vi "MeasureSTARTTime.vi"(8 "error in":errorcluster, 10 "Timeout / ms":u32=1000, 11 "VISA resource name":refnum<visa-resource-name>) -> (0 "error out":errorcluster, 1 "Local time":timestamp, 2 "System time / us":u32=437417, 3 "VISA resource name out":refnum<visa-resource-name>)   [LabVIEW 2017, in "GP22_TDC_Arduinoed.lvlib"]
doc: "Measure the time of arrival of the next pulse at the START input, in milliseconds since the unit was last reset. The counter rolls over every 24 hours."
uses:
  GP22_TDC_Arduinoed.lvlib
  <vilib>/ErrorRing/Error Ring.xnode
  <vilib>/Utility/error.llb/Error Cluster From Error Code.vi
  <vilib>/regexp/Match Regular Expression.xnode
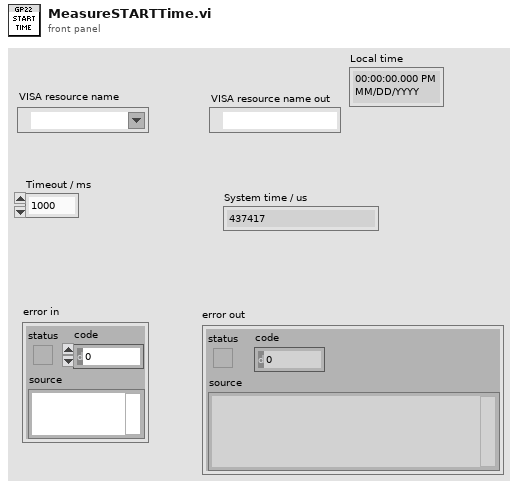
[diagram p1: front panel]
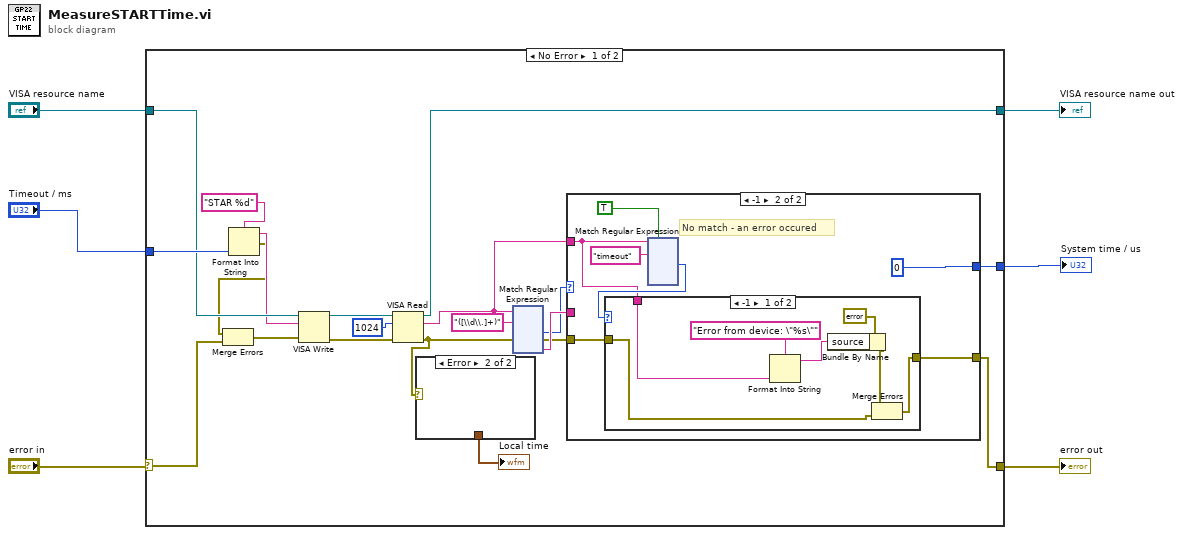
[diagram p0: block diagram]
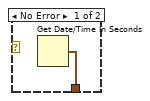
[diagram p2: hidden frame]
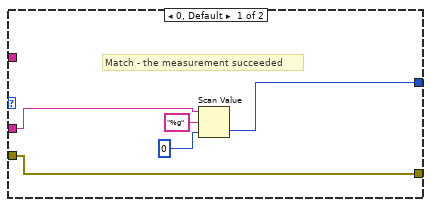
[diagram p3: hidden frame]
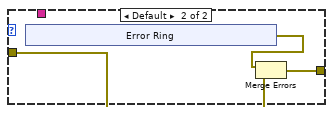
[diagram p4: hidden frame]
diagram:
  n1 = case shown="No Error" "error in" {
    selector: "error in" -> [w20 w288]
    tunnel: "VISA resource name" -> [w24 w287]
    tunnel: [w16 w287] -> w5
    tunnel: [w15 w288] -> w4
    tunnel: "Timeout / ms" -> [w25 _]
    tunnel: [w14 _] -> w1
    frame No Error {
      n2 = Format Into String(format string="STAR %d", w25) -> (resulting string=w23:string, error out=w21:errorcluster)  [unwired: 2 in]
      n3 = Merge Errors(w21, w20) -> (w22:errorcluster)
      n4 = VISA Write(VISA resource name=w24, write buffer=w23, error in (no error)=w22) -> (VISA resource name out=w18:refnum<visa-resource-name>, error out=w19:errorcluster)  [unwired: 1 out]
      n5 = VISA Read(VISA resource name=w18, byte count=u32 1024, error in (no error)=w19) -> (VISA resource name out=w16:refnum<visa-resource-name>, read buffer=w9:string, error out=w8:errorcluster)  [unwired: 1 out]
      n6 = case shown="Error" w8 {
        tunnel: [w27 _] -> w7
        frame No Error {
          n7 = Get Date/Time In Seconds() -> (seconds since 1Jan1904=w27:timestamp)
        }
        frame Error {
        }
      }
      "Local time" <- w7
      n8 = xnode "Match Regular Expression"("input string"=w9, "regular expression"="([\\d\\.]+)", "error in"=w8) -> ("offset past match"=w11:i32, "error out"=w10:errorcluster, "submatch 1"=w12:string)  [unwired: 3 in, 3 out]
      n9 = case shown="-1" w11 {
        tunnel: w10 -> [w145 w154]
        tunnel: [w145 w155] -> w15
        tunnel: w12 -> [w147 _]
        tunnel: [w146 u32 0] -> w14
        tunnel: w9 -> [_ w149]
        frame 0, Default {
          # "Match - the measurement succeeded"
          n10 = Scan Value(string=w147, format string="%g", default (0 dbl)=u32 0) -> (value=w146:u32)  [unwired: 1 out]
        }
        frame -1 {
          # "No match - an error occured"
          n11 = xnode "Match Regular Expression"("input string"=w149, "regular expression"="timeout", "ignore case? (F)"=TRUE) -> ("offset past match"=w150:i32)  [unwired: 3 in, 5 out]
          n12 = case shown="-1" w150 {
            tunnel: [w159 w165] -> w155
            tunnel: w154 -> [w158 w163]
            tunnel: w149 -> [w156 _]
            frame -1 {
              n13 = Format Into String(format string="Error from device: \"%s\"", w156) -> (resulting string=w161:string)  [unwired: 2 in, 1 out]
              n14 = Bundle By Name(cluster=errorcluster {"status"=TRUE, "code"=5000, "source"=""} ("error constant"), "source"=w161) -> (w160:errorcluster)
              n15 = Merge Errors(w160, w158) -> (w159:errorcluster)
            }
            frame Default {
              n16 = xnode "Error Ring"() -> ("error out"=w164:errorcluster)
              n17 = Merge Errors(w164, w163) -> (w165:errorcluster)
            }
          }
        }
      }
    }
    frame Error {
    }
  }
  "VISA resource name out" <- w5
  "error out" <- w4
  "System time / us" <- w1
